vi "TurnDriveTurn-target.vi"(0 "X":dbl, 1 "Description":string, 2 "Angle":dbl, 5 "Y":dbl, 7 "Max time":dbl, 9 "Face angle?":bool, 11 "Command Info In":T1, 12 "Synchronization":enum16{"Start", "Wait"}(ring)) -> (4 "Outcome":string="foo", 15 "Command Info Out":T1)   [LabVIEW 2015]
doc: "This VI sets the motors to run for a given number of seconds. It optionally synchronizes with the completion of the command."
uses:
  <vilib>/Rock Robotics/WPI/Framework/Command Status Info.ctl
  <vilib>/Rock Robotics/WPI/Framework/Completion Status.ctl
  <vilib>/Rock Robotics/WPI/Framework/Completion Notifier.ctl
  Implementation/Drive Setpoints.ctl
  Implementation/Drive Operations.ctl
panel:
  in  "Position":cluster{"X":dbl, "Y":dbl, "Angle":dbl}
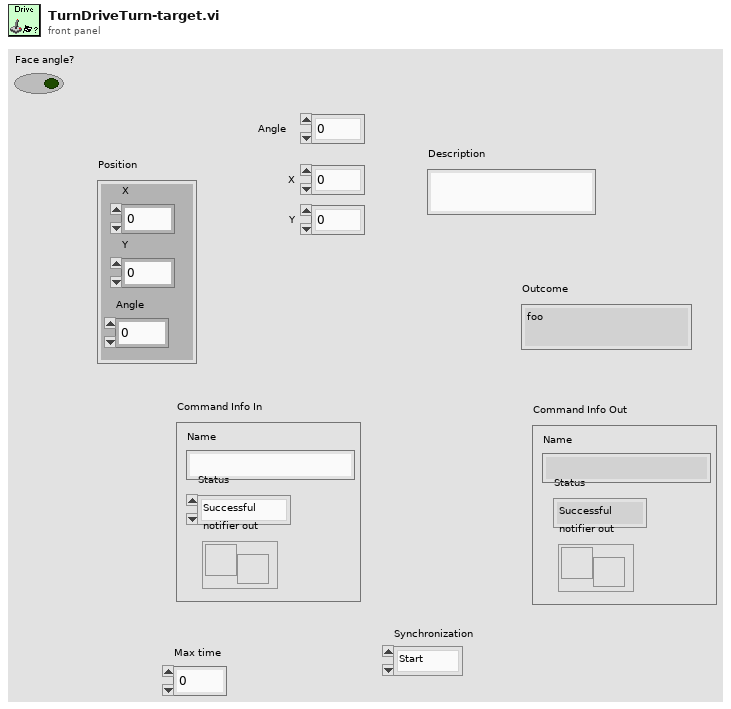
[diagram p1: front panel]
types:
  T1 = typedef "Command Status Info.ctl" = cluster{"Name":string, "Status":T2, "notifier out":T3}
  T2 = typedef "Completion Status.ctl" = enum16{"Successful", "Aborted", "Incomplete"}
  T3 = typedef "Completion Notifier.ctl" = refnum<notifier>
  T4 = typedef "Drive Setpoints.ctl" = cluster{"Operation":T5, "Left Setpoint":dbl, "Right Setpoint":dbl, "Duration":dbl, "Position":cluster{"X":dbl, "Y":dbl, "Angle":dbl}, "Face angle?":bool, "Straight Setpoint":dbl}
  T5 = typedef "Drive Operations.ctl" = enum16{"Reserve", "Read Current", "Immediate", "Turn Drive Turn", "Drive to Target (arc)"}
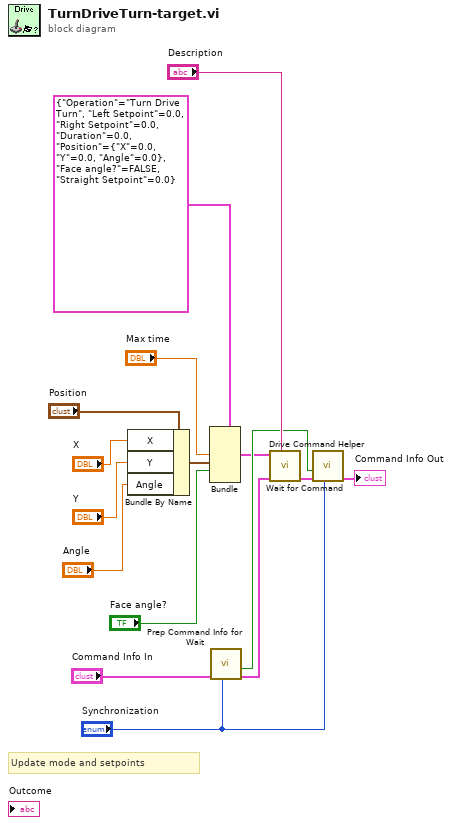
[diagram p0: block diagram]
diagram:
  # "Update mode and setpoints"
  n1 = Bundle By Name(cluster="Position", "X"="X", "Y"="Y", "Angle"="Angle") -> (w4:cluster{"X":dbl, "Y":dbl, "Angle":dbl})
  n2 = Bundle(cluster=T4 {"Operation"=enum."Turn Drive Turn", "Left Setpoint"=0.0, "Right Setpoint"=0.0, "Duration"=0.0, "Position"={"X"=0.0, "Y"=0.0, "Angle"=0.0}, "Face angle?"=FALSE, "Straight Setpoint"=0.0} ("SubSystem Data"), "Duration"="Max time", "Position"=w4, "Face angle?"="Face angle?") -> (w9:T4)  [unwired: 4 in]
  n3 = call <vilib>:"Prep Command Info for Wait.vi"("Synchronication"="Synchronization", "Command Info"="Command Info In") -> ("Command Info"=w13:T1, "Allocated"=w14:bool)  [unwired: 8 in]
  n4 = call "Drive Command Helper.vi"("Description"="Description", "Command Info In"=w13, "SubSystem Data"=w9) -> ("Command Info Out"=w10:T1)  [unwired: 7 in, 1 out]
  n5 = call <vilib>:"Wait for Command.vi"("Synchronication"="Synchronization", "Command Info in"=w10, "Allocated"=w14) -> ("Command Info out"=→"Command Info Out":T1)  [unwired: 8 in]
